vi "Data List.vi"(8 "error in (no error)":errorcluster, 9 "File Path":path, 10 "Table Infor":refnum<class "Data List.lvclass">[](array[class]), 11 "[V]System Tree View in":refnum<class "[V]System Tree View.lvclass">) -> (0 "error out":errorcluster, 3 "[V]System Tree View out":refnum<class "[V]System Tree View.lvclass">)   [LabVIEW 2020, in "[V]System Tree View.lvlib" / "[V]System Tree View.lvclass"]
uses:
  [V]System Tree View.lvclass
  Models/Data List/Data List.lvclass
  [V]System Tree View.lvclass/[V]System Tree View.ctl
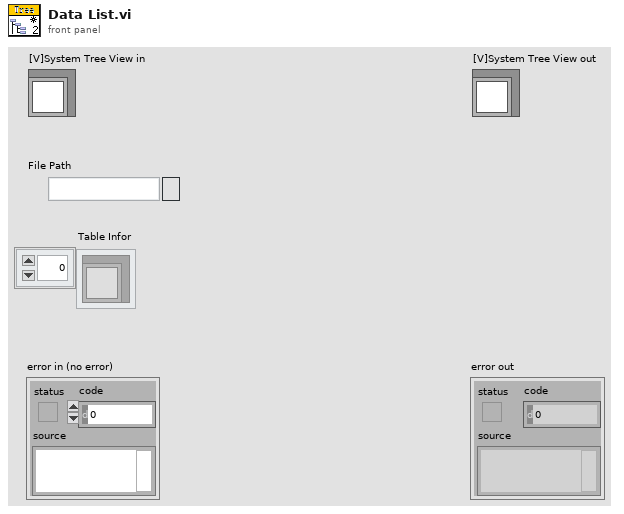
[diagram p1: front panel]
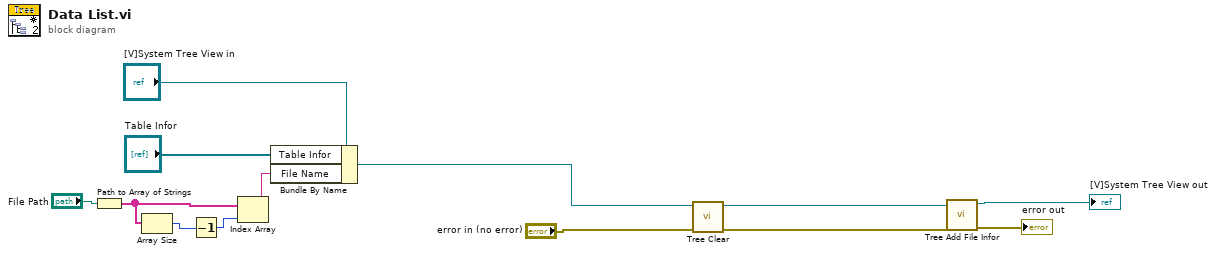
[diagram p0: block diagram]
diagram:
  n1 = Path to Array of Strings(0:"File Path") -> (2:w10:string[])  [unwired: 1 out]
  n2 = Array Size(array=w10) -> (size(s)=w9:i32)
  n3 = Decrement(x=w9) -> (x-1=w8:i32)
  n4 = Index Array(array=w10, index=w8) -> (element=w7:string)
  n5 = Bundle By Name(cluster="[V]System Tree View in", "Table Infor"="Table Infor", "File Name"=w7) -> (w5:refnum<class "[V]System Tree View.lvclass">)
  n6 = call "Tree Clear.vi"("error in (no error)"="error in (no error)", "[V]System Tree View in"=w5) -> ("error out"=w2:errorcluster, "[V]System Tree View out"=w4:refnum<class "[V]System Tree View.lvclass">)  [unwired: 8 in]
  n7 = call "Tree Add File Infor.vi"("error in (no error)"=w2, "[V]System Tree View in"=w4) -> ("error out"=→"error out":errorcluster, "[V]System Tree View out"=→"[V]System Tree View out":refnum<class "[V]System Tree View.lvclass">)  [unwired: 8 in]
